vi "温度采集.vi"() -> ()   [LabVIEW 2013]
uses:
  <vilib>/Instr/_visa.llb/VISA Configure Serial Port (Instr).vi
panel:
  out "工作指示灯":bool
  out "历史数据":dbl(graph)
  in  "停止按钮":bool
  out "温度计":dbl(knob) scale=-20.0..50.0
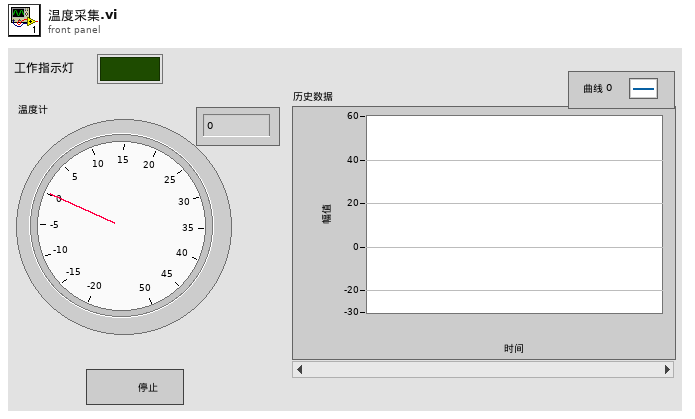
[diagram p1: front panel]
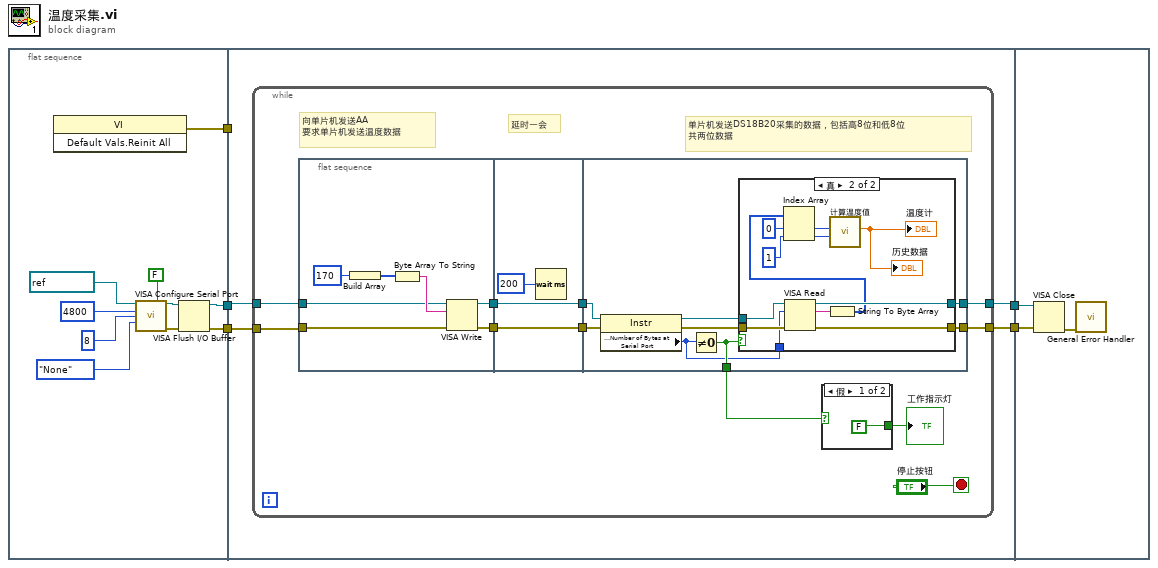
[diagram p0: block diagram]
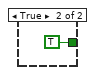
[diagram p2: hidden frame]
diagram:
  n1 = flat-sequence {
    tunnel: [w10] -> w5
    tunnel: [w6] -> w4
    tunnel: [w7] -> w3
    tunnel: w5 -> [_]
    tunnel: w4 -> [w19]
    tunnel: w3 -> [w18]
    tunnel: [w17] -> w2
    tunnel: [w16] -> w1
    tunnel: w2 -> [w65]
    tunnel: w1 -> [w66]
    frame #0 {
      n2 = invoke class="VI" method="Default Vals.Reinit All"() -> (error out=w10:errorcluster)  [unwired: 3 in, 2 out]
      n3 = call-poly "VISA Configure Serial Port"("VISA resource name"=refnum<visa-resource-name> "COM2", "Enable Termination\nChar (T)"=FALSE ("Enable Termination\nChar (T)"), "baud rate (9600)"=u32 4800, "data bits (8)"=u16 8, "parity (0:none)"=enum16{"None", "Odd", "Even", "Mark", "Space"}."None") -> ("VISA resource name out"=w8:refnum<visa-resource-name>, "error out"=w9:errorcluster)  [unwired: 9 in]
      n4 = VISA Flush I/O Buffer(VISA resource name=w8, error in (no error)=w9) -> (VISA resource name out=w6:refnum<visa-resource-name>, error out=w7:errorcluster)  [unwired: 1 in]
    }
    frame #1 {
      n5 = while {
        tunnel: w19 -> [w26]
        tunnel: w18 -> [w25]
        tunnel: [w24] -> w17
        tunnel: [w23] -> w16
        stop <- "停止按钮" stop-if-true
        # "单片机发送DS18B20采集的数据，包括高8位和低8位\n共两位数据"
        # "延时一会"
        # "向单片机发送AA\n要求单片机发送温度数据"
        n6 = flat-sequence {
          tunnel: [w39] -> w30
          tunnel: [w38] -> w29
          tunnel: w26 -> [w34]
          tunnel: w25 -> [w33]
          tunnel: w30 -> [w42]
          tunnel: w29 -> [w41]
          tunnel: [w42] -> w28
          tunnel: [w41] -> w27
          tunnel: w28 -> [w49]
          tunnel: w27 -> [w48]
          tunnel: [w50] -> w23
          tunnel: [w45] -> w24
          tunnel: [w44] -> w20
          frame #0 {
            n7 = Build Array(u8 170) -> (w36:u8[])
            n8 = Byte Array To String(unsigned byte array=w36) -> (string=w35:string)
            n9 = VISA Write(VISA resource name=w34, write buffer=w35, error in (no error)=w33) -> (VISA resource name out=w39:refnum<visa-resource-name>, error out=w38:errorcluster)  [unwired: 1 out]
          }
          frame #1 {
            n10 = Wait (ms)(milliseconds to wait=u32 200 ("等待时间（毫秒）")) -> ()  [unwired: 1 out]
          }
          frame #2 {
            n11 = property class="Instr"(reference=w49, error in=w48) -> (reference out=w47:refnum<visa-resource-name>, error out=w46:errorcluster, "Serial Settings:Number of Bytes at Serial Port"=w43:u32)
            n12 = Not Equal To 0?(x=w43) -> (x != 0?=w44:bool)
            n13 = case shown="真" w44 {
              tunnel: [w51 w64] -> w50
              tunnel: w47 -> [w52 w63]
              tunnel: w46 -> [w51 w62]
              tunnel: [w52 w61] -> w45
              tunnel: w43 -> [_ w53]
              frame False {
              }
              frame True {
                n14 = VISA Read(VISA resource name=w63, byte count=w53, error in (no error)=w62) -> (VISA resource name out=w61:refnum<visa-resource-name>, read buffer=w60:string, error out=w64:errorcluster)  [unwired: 1 out]
                n15 = String To Byte Array(string=w60) -> (unsigned byte array=w57:u8[])
                n16 = Index Array(array=w57, index #1=0 ("索引"), index #2=1 ("索引")) -> (element #1=w56:u8, element #2=w55:u8)
                n17 = call "计算温度值.vi"("数值L"=w55, "数值H"=w56) -> ("温度"=→"历史数据" →"温度计":dbl)  [unwired: 9 in]
              }
            }
          }
        }
        n18 = case shown="假" w20 {
          tunnel: [FALSE ("工作指示灯") TRUE ("工作指示灯")] -> w21
          frame False {
          }
          frame True {
          }
        }
        "工作指示灯" <- w21
      }
    }
    frame #2 {
      n19 = VISA Close(VISA resource name=w65, error in (no error)=w66) -> (error out=w67:errorcluster)
      n20 = call <vilib>:"General Error Handler.vi"("error in (no error)"=w67) -> ()  [unwired: 10 in, 5 out]
    }
  }
